vi "OpenClose-Item.vi"(8 "error in (no error)":errorcluster, 9 "Open?":bool, 10 "Tag":string, 11 "TreeDirectoryExt in":refnum<class "TreeDirectoryExt.lvclass">) -> (0 "error out":errorcluster, 3 "TreeDirectoryExt out":refnum<class "TreeDirectoryExt.lvclass">)   [LabVIEW 2026, in "TreeDirectoryExt.lvclass"]
doc: "Expands or closes a node in the tree control.\n\nQControl Class wrapper around the <b>Open/Close : Item Method</b>.\n<b> </b> <b> </b>\n©2016 Q Software Innovations, LLC (QSI)\nwritten by Quentin Alldredge\nproduced in LabVIEW 2015\n\nsupport@qsoftwareinnovations.com\nwww.qsoftwareinnovations.com\n\nAll rights reserved.\n\nRedistribution and use in source and binary forms, with or without modification, are permitted provided that the following conditions are met:\n\n * Redistributions of source code must retain the above copyright notice, this list of conditions and the following disclaimer.\n * Redistributions in binary form must reproduce the above copyright notice, this list of conditions and the following disclaimer in the documentation and/or other materials provided with the distribution.\n * Neither the name of Q Software Innovations, LLC. nor the names of its contributors may be used to endorse or promote products derived from this software without specific prior written permission.\n\nTHIS SOFTWARE IS PROVIDED BY THE COPYRIGHT HOLDERS AND CONTRIBUTORS \"AS IS\" AND ANY EXPRESS OR IMPLIED WARRANTIES, INCLUDING, BUT NOT LIMITED TO, THE IMPLIED WARRANTIES OF MERCHANTABILITY AND FITNESS FOR A PARTICULAR PURPOSE ARE DISCLAIMED. IN NO EVENT SHALL THE COPYRIGHT OWNER OR CONTRIBUTORS BE LIABLE FOR ANY DIRECT, INDIRECT, INCIDENTAL, SPECIAL, EXEMPLARY, OR CONSEQUENTIAL DAMAGES (INCLUDING, BUT NOT LIMITED TO, PROCUREMENT OF SUBSTITUTE GOODS OR SERVICES; LOSS OF USE, DATA, OR PROFITS; OR BUSINESS INTERRUPTION) HOWEVER CAUSED AND ON ANY THEORY OF LIABILITY, WHETHER IN CONTRACT, STRICT LIABILITY, OR TORT (INCLUDING NEGLIGENCE OR OTHERWISE) ARISING IN ANY WAY OUT OF THE USE OF THIS SOFTWARE, EVEN IF ADVISED OF THE POSSIBILITY OF SUCH DAMAGE."
uses:
  TreeDirectoryExt.lvclass
  <vilib>/QSI/QControls/QControl Classes/TreeControl/TreeControl.lvclass
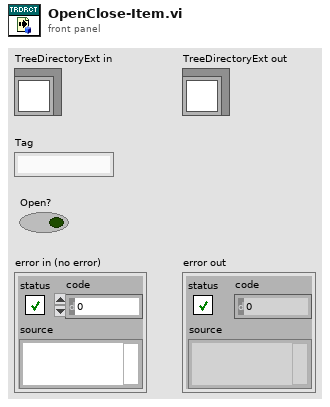
[diagram p1: front panel]
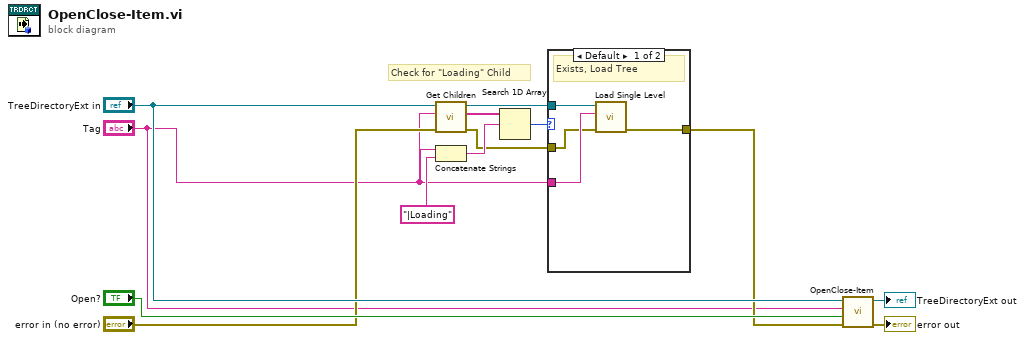
[diagram p0: block diagram]
diagram:
  # "Check for \"Loading\" Child"
  n1 = call <vilib>:"Get Children.vi"("error in (no error)"="error in (no error)", "Tag"="Tag", "Tree in"="TreeDirectoryExt in") -> ("error out"=w5:errorcluster, "ChildrenTags[]"=w9:string[], "Tree out"=w6:refnum<class "TreeDirectoryExt.lvclass">)  [unwired: 6 in]
  n2 = Concatenate Strings("Tag", "|Loading" ("string")) -> (w8:string)
  n3 = Search 1D Array(1D array=w9, element=w8) -> (index of element=w7:i32)  [unwired: 1 in]
  n4 = case shown="Default" w7 {
    tunnel: w6 -> [w17 _]
    tunnel: "Tag" -> [w16 _]
    tunnel: w5 -> [w15 w18]
    tunnel: [w14 w18] -> w3
    frame Default {
      # "Exists, Load Tree"
      n5 = call "Load Single Level.vi"("error in (no error)"=w15, "Tag"=w16, "TreeDirectory in"=w17) -> ("error out"=w14:errorcluster)  [unwired: 7 in, 1 out]
    }
    frame -1 {
      # "DNE, Do Nothing"
    }
  }
  n6 = call-parent "OpenClose-Item.vi"("error in (no error)"=w3, "Open?"="Open?", "Tag"="Tag", "TreeControl in"="TreeDirectoryExt in") -> ("error out"=→"error out":errorcluster, "TreeControl out"=→"TreeDirectoryExt out":refnum<class "TreeDirectoryExt.lvclass">)  [unwired: 6 in]
